vi "参数输出转换.vi"(11 "Registers":u16[](array[numeric])) -> (3 "参数":T1={"低压报警阈值 V"=21.0, "低压报警解除阈值 V"=21.0, "高温报警阈值 ℃"=50.0, "高温报警解除阈值 ℃"=50.0, "湿度报警阈值 %"=95.0, "湿度报警解除阈值 %"=95.0, "冷却风扇启动阈值 ℃"=35.0, "冷却风扇停止阈值 ℃"=30.0})   [LabVIEW 2016, in "环境动力单元.lvlib"]
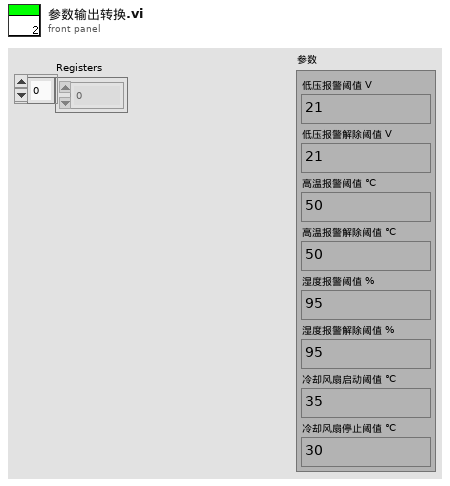
[diagram p1: front panel]
types:
  T1 = cluster{"低压报警阈值 V":dbl, "低压报警解除阈值 V":dbl, "高温报警阈值 ℃":dbl, "高温报警解除阈值 ℃":dbl, "湿度报警阈值 %":dbl, "湿度报警解除阈值 %":dbl, "冷却风扇启动阈值 ℃":dbl, "冷却风扇停止阈值 ℃":dbl}
  T2 = cluster{"Registers[0]":u16, "Registers[1]":u16, "Registers[2]":u16, "Registers[3]":u16, "Registers[4]":u16, "Registers[5]":u16, "Registers[6]":u16, "Registers[7]":u16}
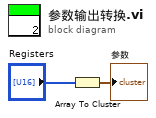
[diagram p0: block diagram]
diagram:
  n1 = Array To Cluster(array="Registers") -> (cluster=→"参数":T2)
